vi "Main.vi"() -> ()   [LabVIEW 2020]
doc: "Use this template to build a simple state machine design pattern. Each state executes code and determines which state to transition to."
uses:
  controls/State.ctl
  controls/Data.ctl
  controls/LH Data.ctl
  controls/Pump Data.ctl
  <instrlib>/Eurotherm 32xx Series/Eurotherm 32xx Series.lvlib
  <instrlib>/rheodyne/rheodyne.lvlib
panel:
  in  "High Level Tab":T1(tab)
  in  "VISA Selection Valve":refnum<visa-resource-name>
  in  "ID":u16=22
  in  "VISA Detector":refnum<visa-resource-name>
  out "Temperature":dbl
  out "Flowrate":dbl
  in  "VISA Sample Loop":refnum<visa-resource-name>
  in  "VISA Reactor":refnum<visa-resource-name>
  in  "Reservoir Level":dbl
  in  "VISA Isolation":refnum<visa-resource-name>
  in  "VISA Multiway":refnum<visa-resource-name>
  in  "VISA Gilson":refnum<visa-resource-name>
  in  "VISA Solvent Pump":refnum<visa-resource-name>
  in  "Solvents":dbl[](array[numeric])
  in  "Equipment Tab":T2(tab)
  in  "Tab LH":enum32{"Manual", "Automated"}(tab)
  in  "Sample LH":bool
  in  "Volume Array":u32[](array[numeric])
  in  "Y Array":u32[](array[numeric])
  in  "X Array":u32[](array[numeric])
  in  "Needle LH":bool
  in  "Move LH":bool
  in  "Z Position":u32
  in  "Y Position":u32
  in  "X Position":u32
  in  "Calibration R-squared":dbl[](array[numeric])
  in  "Calibration Coefficients":dbl[][](array[numeric])
  in  "Calibrate":bool
  out "Process Value - Chart":sgl(graph) caption="Waveform Chart - Light"
  in  "Controller  Mode":enum16{"Auto", "Manual"}(ring)
  in  "Keylock":T3(ring)
  in  "Temperature \nSetpoint":dbl=15.0
  out "Stable Temp?":bool
  in  "TC Noise Tolerance":dbl=0.1
  out "Current \nTemperature":dbl
  in  "# Samples to average":i32=20
  in  "Sample time (ms)":u32=100
  out "Alarms Output":bool
  out "New Alarms":bool
  in  "Sampling time (ms)":u16
  in  "Monitor":bool
  in  "Set Wavelength (nm)":u16
  out "Waveform Chart - Light":dbl(graph)
  out "Absorbance":dbl
  in  "Stop Button":bool
  # "Movement"
  # "Recipe"
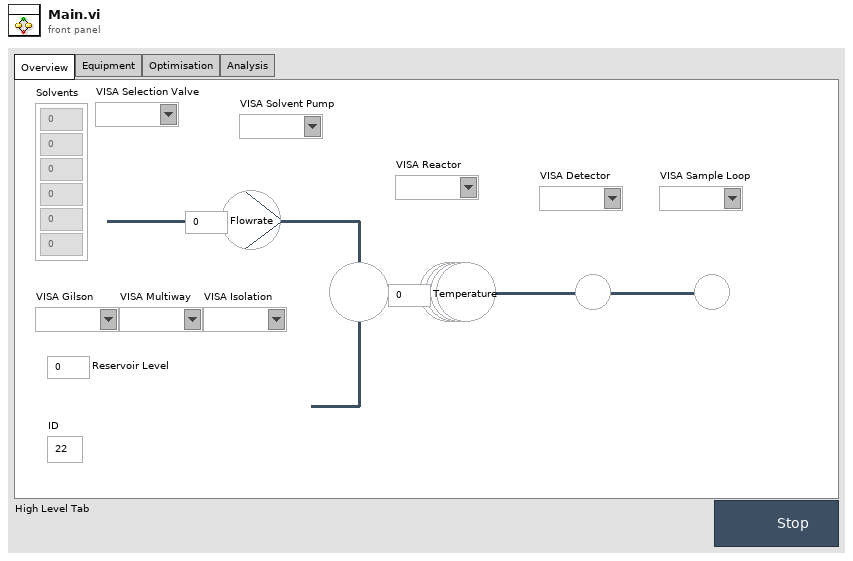
[diagram p1: front panel]
types:
  T1 = enum32{"Overview", "Equipment", "Optimisation", "Analysis"}
  T2 = enum32{"Liquid Handler", "Pump", "Reactor", "Detector"}
  T3 = enum16{"None", "All", "Edit", "mod", "mAn", "Stby", "tmr"}
  T4 = cluster{"Baud Rate (19200)":u32, "Parity (0: None)":u16, "Break Length (0)":u16}
  T5 = typedef "Data.ctl" = cluster{"Liquid Handler":T6, "Pump":T7, "VISA Selection Valve":refnum<visa-resource-name>}
  T6 = typedef "LH Data.ctl" = cluster{"X Position":u32, "Y Position":u32, "Z Position":u32, "Recipe":cluster{"X Array":u32[], "Y Array":u32[], "Volume Array":u32[]}, "VISA Gilson":refnum<visa-resource-name>, "VISA Multiway":refnum<visa-resource-name>, "VISA Isolation":refnum<visa-resource-name>, "Move LH":bool, "Needle LH":bool, "Sample LH":bool}
  T7 = typedef "Pump Data.ctl" = cluster{"Calibrated":bool, "Flowrate":dbl, "VISA Pump":refnum<visa-resource-name>, "Calibration Coefficients":dbl[][], "Solvents":dbl[]}
  T8 = typedef "State.ctl" = enum16{"Initialize", "Wait for Event", "Manual LH", "Manual Valve", "Calibrate Pump", "Exit"}
  T9 = cluster{"X Array":u32[], "Y Array":u32[], "Volume Array":u32[]}
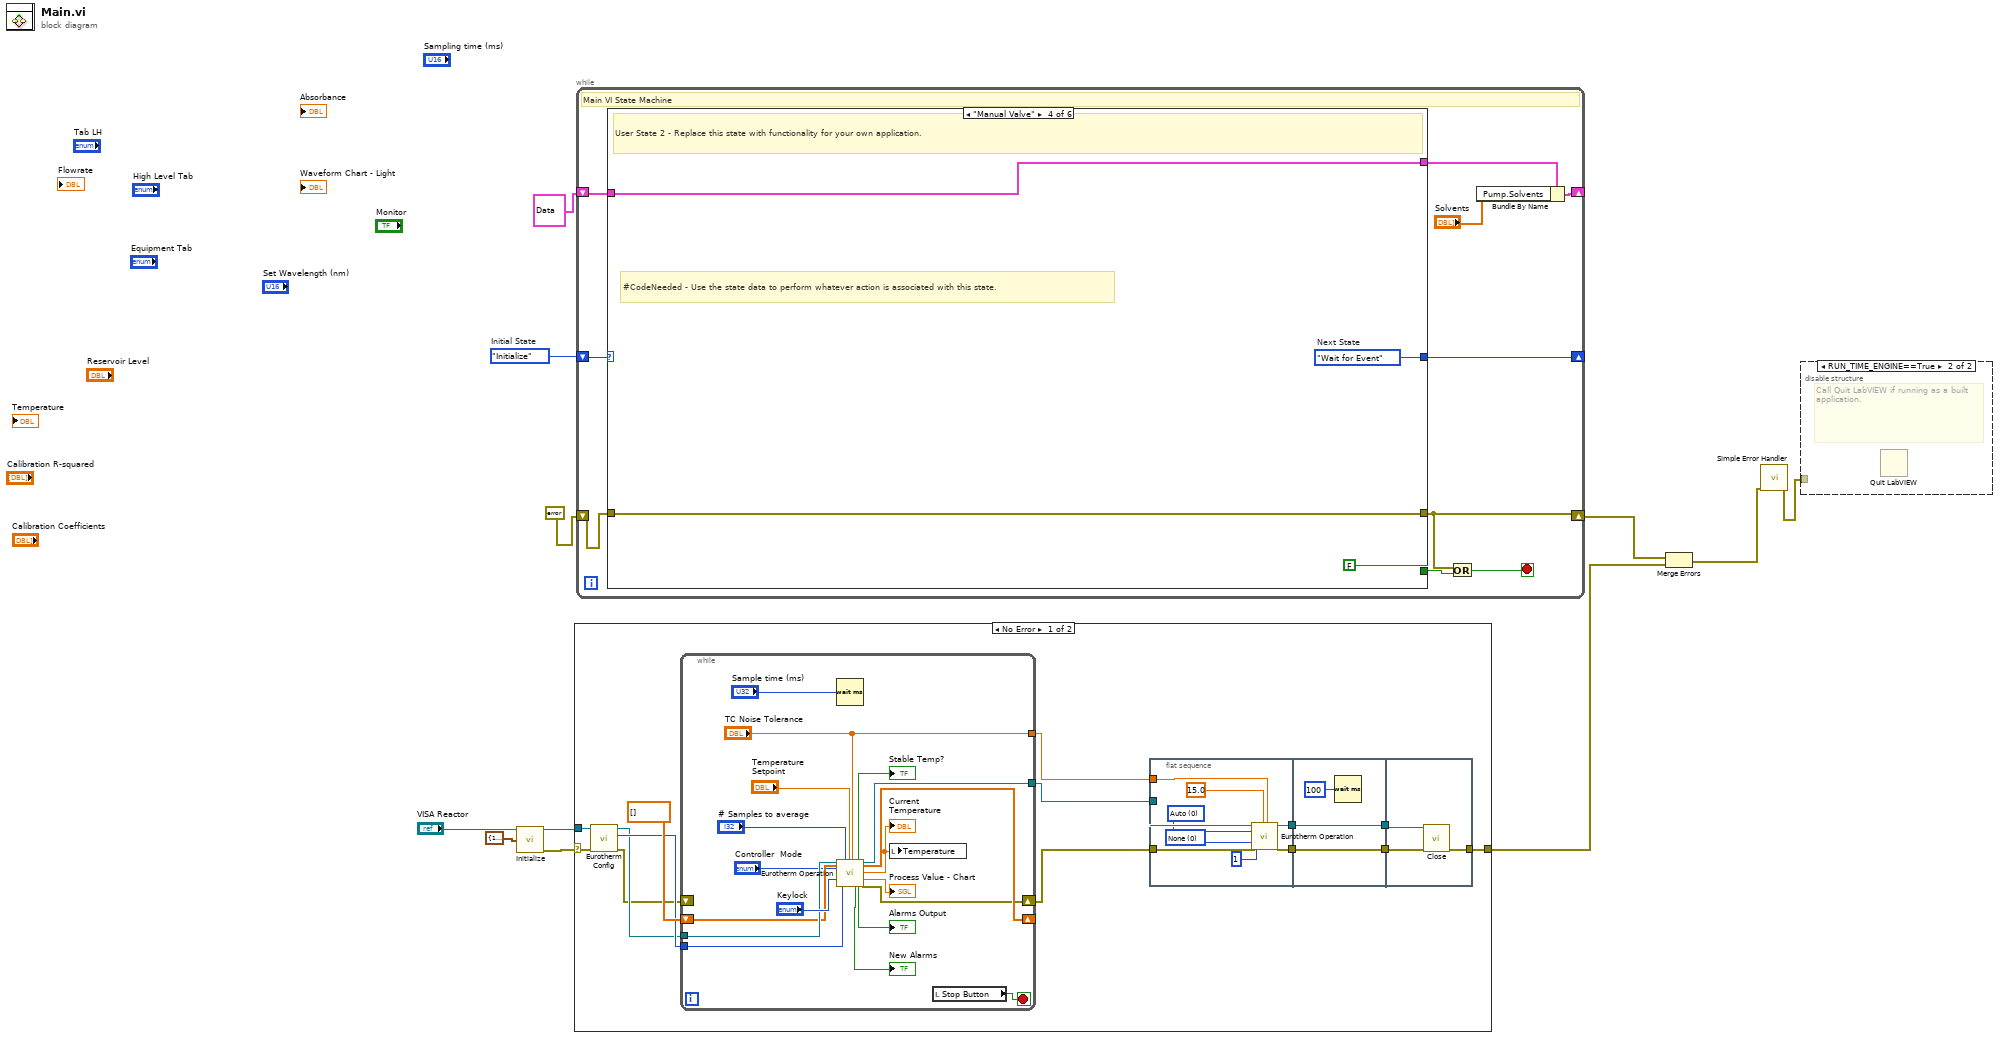
[diagram p0: block diagram]
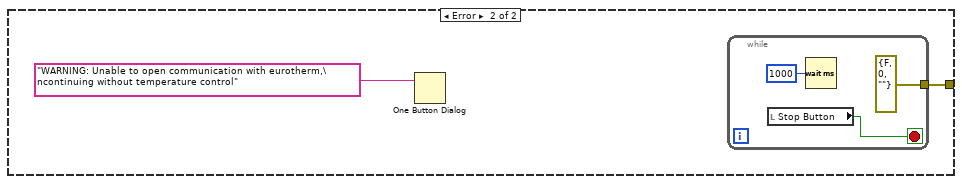
[diagram p2: hidden frame]
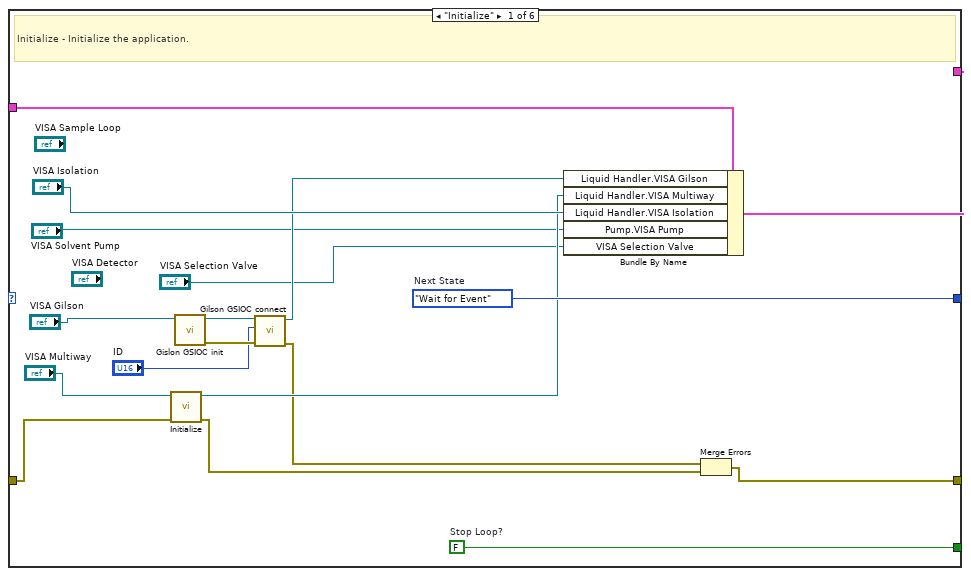
[diagram p4: hidden frame]
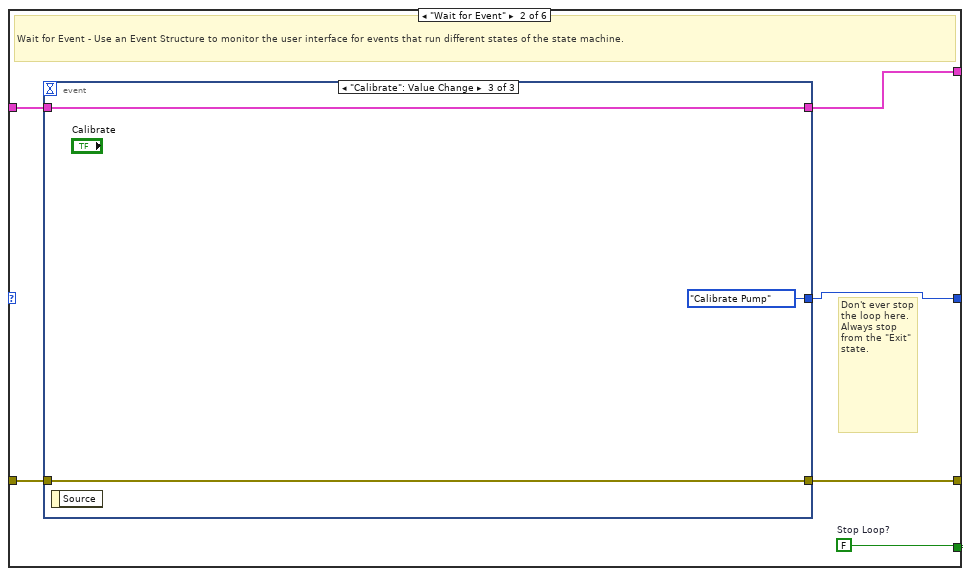
[diagram p5: hidden frame]
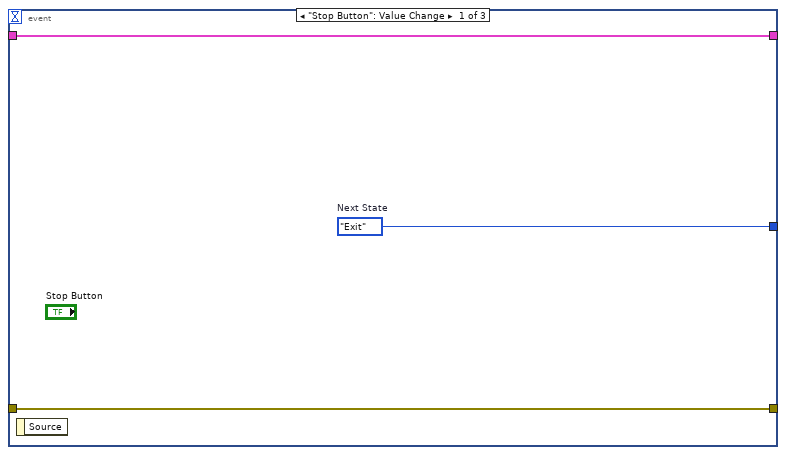
[diagram p6: hidden frame]
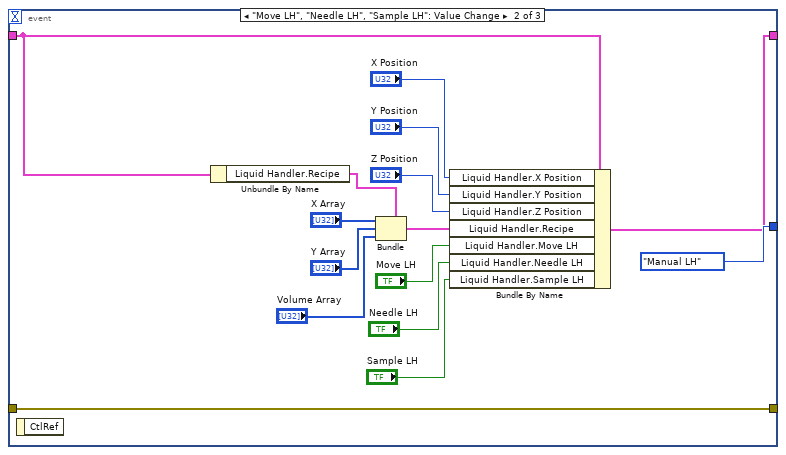
[diagram p7: hidden frame]
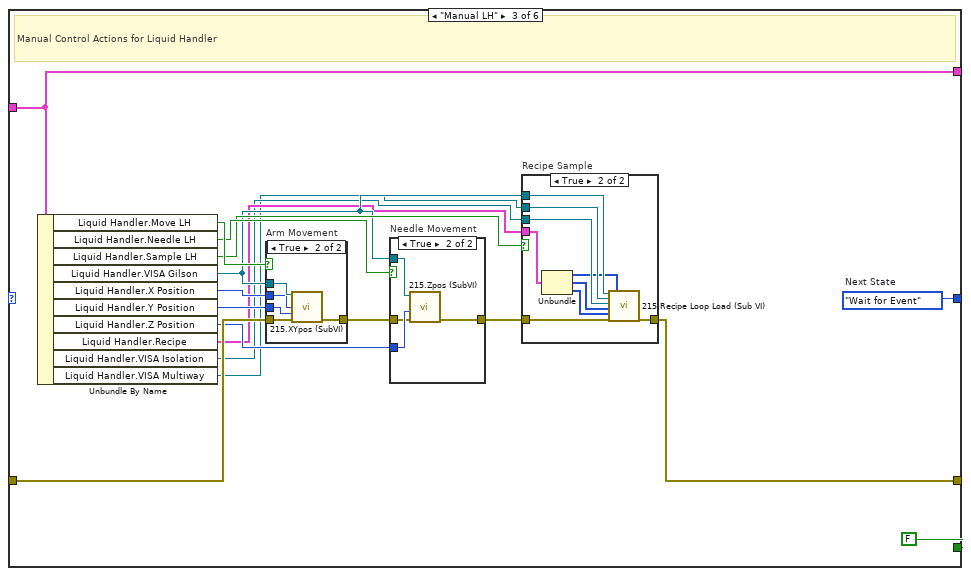
[diagram p8: hidden frame]
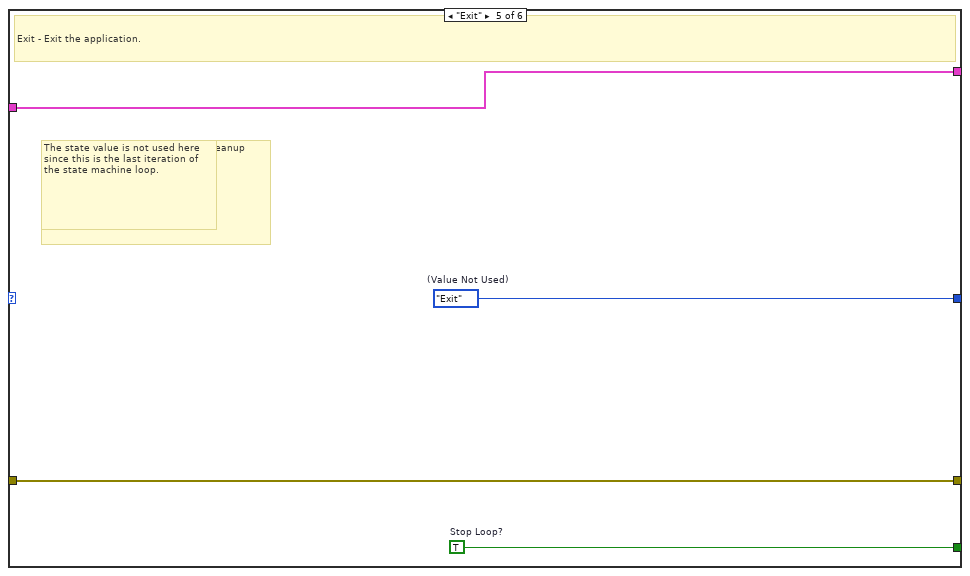
[diagram p12: hidden frame]
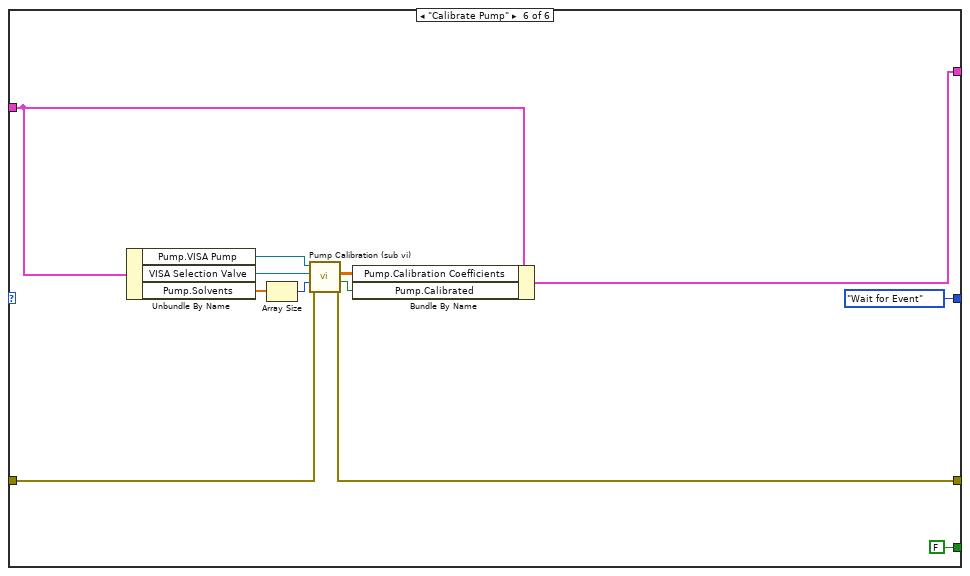
[diagram p13: hidden frame]
diagram:
  w11 = State."Initialize"  # Initial State
  n1 = call <instrlib>:"Initialize.vi"("VISA resource name"="VISA Reactor", "Serial Configuration"=T4 {"Baud Rate (19200)"=19200, "Parity (0: None)"=0, "Break Length (0)"=20}) -> ("VISA resource name out"=w2:refnum<visa-resource-name>, "error out"=w1:errorcluster)  [unwired: 12 in]
  n2 = case shown="No Error" w1 {
    selector: w1 -> [w13 _]
    tunnel: [w17 w60] -> w4
    tunnel: w2 -> [w16 _]
    frame No Error {
      n3 = call "Eurotherm Config.vi"("error in (no error)"=w13, "VISA Refnum in"=w16) -> ("error out"=w12:errorcluster, "Unit Address (1)"=w15:u8, "VISA Refnum out"=w14:refnum<visa-resource-name>)  [unwired: 7 in]
      n4 = while {
        tunnel: w15 -> [w54]
        tunnel: [w55] -> w20
        tunnel: ["TC Noise Tolerance"] -> w21
        tunnel: w14 -> [w52]
        shift-right: [w43] -> w18
        shift-left: w12 -> [_]
        shift-right: [w51] -> _
        shift-left: sgl[] [] ("Array out") -> [w50]
        stop <- w42 stop-if-true
        n5 = Wait (ms)(milliseconds to wait="Sample time (ms)") -> ()  [unwired: 1 out]
        n6 = call "Eurotherm Operation.vi"("VISA Refnum in"=w52, "Array in"=w50, "Controller  Mode in"="Controller  Mode", "Keylock in"="Keylock", "Unit Address (1)"=w54, "# Samples to average in"="# Samples to average", "Setpoint Temperature (°C) in"="Temperature \nSetpoint", "Noise tolerance (°C)"="TC Noise Tolerance") -> ("New ALARM !"=→"New Alarms":bool, "Reached set temp and ready?"=→"Stable Temp?":bool, "Alarm Output"=→"Alarms Output":bool, "VISA Refnum out"=w55:refnum<visa-resource-name>, "Array out"=w51:sgl[], "Curent Temperature (°C)"=w41:sgl, "Process Value - Chart"=→"Process Value - Chart":sgl, "error out"=w43:errorcluster)  [unwired: 12 in]
        "Current \nTemperature" <- w41
        n7 = local write "Temperature"(w41) -> ()
        n8 = local read "Stop Button"() -> (w42:bool)
      }
      n9 = flat-sequence {
        tunnel: w21 -> [w33]
        tunnel: w20 -> [w32]
        tunnel: w18 -> [w31]
        tunnel: [w34] -> w25
        tunnel: [w26] -> w24
        tunnel: w25 -> [w37]
        tunnel: [w37] -> w23
        tunnel: w24 -> [w36]
        tunnel: [w36] -> w22
        tunnel: w23 -> [w39]
        tunnel: w22 -> [w40]
        tunnel: [w38] -> w17
        frame #0 {
          w27 = u8 0 items=["Auto", "Manual"] ("Controller  Mode in")
          w29 = u8 0 items=["None", "All", "Edit", "mod", "mAn", "Stby", "tmr"] ("Keylock in")
          n10 = call "Eurotherm Operation.vi"("VISA Refnum in"=w32, "Controller  Mode in"=w27, "Keylock in"=w29, "error in (no error)"=w31, "Unit Address (1)"=u8 1, "Setpoint Temperature (°C) in"=15.0, "Noise tolerance (°C)"=w33) -> ("VISA Refnum out"=w34:refnum<visa-resource-name>, "error out"=w26:errorcluster)  [unwired: 13 in, 6 out]
        }
        frame #1 {
          n11 = Wait (ms)(milliseconds to wait=u32 100) -> ()  [unwired: 1 out]
        }
        frame #2 {
          n12 = call <instrlib>:"Close.vi"("VISA resource name"=w39, "error in (no error)"=w40) -> ("error out"=w38:errorcluster)  [unwired: 13 in]
        }
      }
    }
    frame Error {
      n13 = One Button Dialog(message="WARNING: Unable to open communication with eurotherm,\ncontinuing without temperature control") -> ()  [unwired: 1 in, 1 out]
      n14 = while {
        tunnel: [errorcluster {"status"=FALSE, "code"=0, "source"=""} ("error out")] -> w60
        stop <- w62 stop-if-true
        n15 = local read "Stop Button"() -> (w62:bool)
        n16 = Wait (ms)(milliseconds to wait=u32 1000) -> ()  [unwired: 1 out]
      }
    }
  }
  n17 = while {
    shift-right: [w72] -> _
    shift-left: w11 -> [w73]
    shift-right: [w65] -> _
    shift-left: T5 {"Liquid Handler"={"X Position"=0, "Y Position"=0, "Z Position"=0, "Recipe"={"X Array"=[], "Y Array"=[], "Volume Array"=[]}, "VISA Gilson"="", "VISA Multiway"="", "VISA Isolation"="", "Move LH"=FALSE, "Needle LH"=FALSE, "Sample LH"=FALSE}, "Pump"={"Calibrated"=FALSE, "Flowrate"=0.0, "VISA Pump"="", "Calibration Coefficients"=[], "Solvents"=[]}, "VISA Selection Valve"=""} ("Data") -> [w71]
    shift-right: [w67] -> w5
    shift-left: errorcluster {"status"=FALSE, "code"=0, "source"=""} ("error constant") -> [w70]
    stop <- w68 stop-if-true
    # "Main VI State Machine"
    n18 = case shown="\"Manual Valve\"" w73 {
      tunnel: [w91 w97 w135 w160 w164 State."Wait for Event" ("(Value Not Used)")] -> w72
      tunnel: [w90 w96 FALSE ("Stop Loop?") FALSE ("Stop Loop?") w162 FALSE ("Stop Loop?")] -> w69
      tunnel: w71 -> [w89 w95 w130 w158 w163 w175]
      tunnel: [w88 w94 w130 w158 w163 w174] -> w66
      tunnel: w70 -> [w84 w93 w129 w157 w161 w170]
      tunnel: [w78 w92 w126 w157 w161 w169] -> w67
      frame "Initialize" {
        w90 = FALSE  # Stop Loop?
        w91 = State."Wait for Event"  # Next State
        # "Initialize - Initialize the application."
        n19 = call <instrlib>:"Initialize.vi"("error in (no error)"=w84, "VISA resource name"="VISA Multiway") -> ("error out"=w76:errorcluster, "VISA resource name out"=w85:refnum<visa-resource-name>)  [unwired: 8 in]
        n20 = call <instrlib>:"Gislon GSIOC init.vi"("VISA resource name"="VISA Gilson") -> ("error out"=w82:errorcluster, "VISA resource name out"=w83:refnum<visa-resource-name>)  [unwired: 9 in]
        n21 = call <instrlib>:"Gilson GSIOC connect.vi"("error in (no error)"=w82, "ID (1)"="ID", "VISA resource name"=w83) -> ("error out"=w77:errorcluster, "VISA resource name"=w80:refnum<visa-resource-name>)  [unwired: 6 in, 1 out]
        n22 = Bundle By Name(cluster=w89, "Liquid Handler.VISA Gilson"=w80, "Liquid Handler.VISA Multiway"=w85, "Liquid Handler.VISA Isolation"="VISA Isolation", "Pump.VISA Pump"="VISA Solvent Pump", "VISA Selection Valve"="VISA Selection Valve") -> (w88:T5)
        n23 = Merge Errors(w77, w76) -> (w78:errorcluster)
      }
      frame "Wait for Event" {
        w96 = FALSE  # Stop Loop?
        # "Don't ever stop the loop here. Always stop from the \"Exit\" state."
        # "Wait for Event - Use an Event Structure to monitor the user interface for events that run different states of the state machine."
        n24 = event shown="[2] \"Calibrate\": Value Change" {
          selector: _ -> [_ _ _]
          dyn-events: _ -> [_ _ _]
          timeout: _ -> [_ _ _]
          tunnel: [w100 State."Manual LH" ("Next State") State."Calibrate Pump" ("Next State")] -> w97
          tunnel: w95 -> [w99 w112 w118]
          tunnel: [w99 w113 w118] -> w94
          tunnel: w93 -> [w98 w115 w117]
          tunnel: [w98 w115 w117] -> w92
          event "Stop Button": Value Change {
            w100 = State."Exit"  # Next State
            n25 = event-data() -> ()  [unwired: 1 in, 1 out]
          }
          event "Move LH", "Needle LH", "Sample LH": Value Change {
            n26 = event-data() -> ()  [unwired: 1 in, 1 out]
            n27 = Unbundle By Name(w112) -> ("Liquid Handler.Recipe"=w111:T9)
            n28 = Bundle(cluster=w111, "X Array"="X Array", "Y Array"="Y Array", "Volume Array"="Volume Array") -> (w104:T9)
            n29 = Bundle By Name(cluster=w112, "Liquid Handler.X Position"="X Position", "Liquid Handler.Y Position"="Y Position", "Liquid Handler.Z Position"="Z Position", "Liquid Handler.Recipe"=w104, "Liquid Handler.Move LH"="Move LH", "Liquid Handler.Needle LH"="Needle LH", "Liquid Handler.Sample LH"="Sample LH") -> (w113:T5)
          }
          event "Calibrate": Value Change {
            n30 = event-data() -> ()  [unwired: 1 in, 1 out]
          }
        }
      }
      frame "Manual LH" {
        w135 = State."Wait for Event"  # Next State
        # "Manual Control Actions for Liquid Handler"
        n31 = Unbundle By Name(w130) -> ("Liquid Handler.Move LH"=w133:bool, "Liquid Handler.Needle LH"=w132:bool, "Liquid Handler.Sample LH"=w131:bool, "Liquid Handler.VISA Gilson"=w125:refnum<visa-resource-name>, "Liquid Handler.X Position"=w124:u32, "Liquid Handler.Y Position"=w123:u32, "Liquid Handler.Z Position"=w122:u32, "Liquid Handler.Recipe"=w121:T9, "Liquid Handler.VISA Isolation"=w120:refnum<visa-resource-name>, "Liquid Handler.VISA Multiway"=w119:refnum<visa-resource-name>)
        n32 = case "Arm Movement" shown="True" w133 {
          tunnel: w129 -> [w151 w156]
          tunnel: [w151 w155] -> w128
          tunnel: w125 -> [_ w154]
          tunnel: w124 -> [_ w153]
          tunnel: w123 -> [_ w152]
          frame False {
          }
          frame True {
            n33 = call "215.XYpos (SubVI).vi"("VISA resource name"=w154, "X"=w153, "Y"=w152, "error in (no error)"=w156) -> ("error out"=w155:errorcluster)  [unwired: 8 in, 3 out]
          }
        }
        n34 = case "Needle Movement" shown="True" w132 {
          tunnel: w128 -> [w146 w148]
          tunnel: [w146 w147] -> w127
          tunnel: w125 -> [_ w150]
          tunnel: w122 -> [_ w149]
          frame False {
          }
          frame True {
            n35 = call "215.Zpos (SubVI).vi"("error in (no error)"=w148, "Z"=w149, "VISA resource name"=w150) -> ("error out"=w147:errorcluster)  [unwired: 5 in, 3 out]
          }
        }
        n36 = case "Recipe Sample" shown="True" w131 {
          tunnel: w127 -> [w136 w138]
          tunnel: [w136 w137] -> w126
          tunnel: w125 -> [_ w143]
          tunnel: w121 -> [_ w142]
          tunnel: w120 -> [_ w145]
          tunnel: w119 -> [_ w144]
          frame False {
          }
          frame True {
            n37 = Unbundle(w142) -> ("X Array"=w141:u32[], "Y Array"=w140:u32[], "Volume Array"=w139:u32[])
            n38 = call "215.Recipe Loop Load (Sub VI).vi"("VISA Gilson"=w143, "VISA Multi-position Valve"=w144, "VISA Isolation Valve"=w145, "Y Position List"=w140, "Volume List"=w139, "error in (no error)"=w138, "X Position List"=w141) -> ("error out"=w137:errorcluster)  [unwired: 10 in, 2 out]
          }
        }
      }
      frame "Manual Valve" {
        w160 = State."Wait for Event"  # Next State
        # "#CodeNeeded - Use the state data to perform whatever action is associated with this state."
        # "User State 2 - Replace this state with functionality for your own application."
      }
      frame "Exit" {
        w162 = TRUE  # Stop Loop?
        w164 = State."Exit"  # (Value Not Used)
        # "#CodeNeeded - Add any required cleanup code here.\nCorrect shutdown procedure"
        # "The state value is not used here since this is the last iteration of the state machine loop."
        # "Exit - Exit the application."
      }
      frame "Calibrate Pump" {
        n39 = Unbundle By Name(w175) -> ("Pump.VISA Pump"=w173:refnum<visa-resource-name>, "VISA Selection Valve"=w172:refnum<visa-resource-name>, "Pump.Solvents"=w165:dbl[])
        n40 = Array Size(array=w165) -> (size(s)=w171:i32)
        n41 = call "Pump Calibration (sub vi).vi"("error in (no error)"=w170, "No. Solvents"=w171, "VISA Valve"=w172, "VISA Pump"=w173) -> ("error out"=w169:errorcluster, "Calibrated"=w167:bool, "Polynomial Coefficients"=w168:dbl[][])  [unwired: 5 in]
        n42 = Bundle By Name(cluster=w175, "Pump.Calibration Coefficients"=w168, "Pump.Calibrated"=w167) -> (w174:T5)
      }
    }
    n43 = Or(x=w67, y=w69) -> (x .or. y?=w68:bool)
    n44 = Bundle By Name(cluster=w66, "Pump.Solvents"="Solvents") -> (w65:T5)
  }
  n45 = Merge Errors(w5, w4) -> (w3:errorcluster)
  n46 = call <vilib>:"Simple Error Handler.vi"("error in (no error)"=w3) -> ("error out"=w8:errorcluster)  [unwired: 4 in, 4 out]
  n47 = disable-structure shown="RUN_TIME_ENGINE==True" {
    disable-tunnel: w8 -> [_ _]
    frame condition #0 (active) {
    }
    frame condition #1 {
      # "Call Quit LabVIEW if running as a built application."
      n48 = Quit LabVIEW() -> ()  [unwired: 1 in]
    }
  }
